vi "Position First Tab Button.vi"(7 "TabCtl Refnum":refnum<vi>, 8 "error in (no error)":errorcluster, 11 "Button Ref":refnum<vi>) -> (0 "error out":errorcluster)   [LabVIEW 2014]
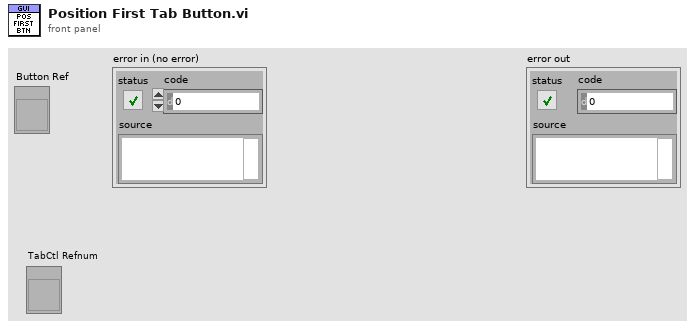
[diagram p1: front panel]
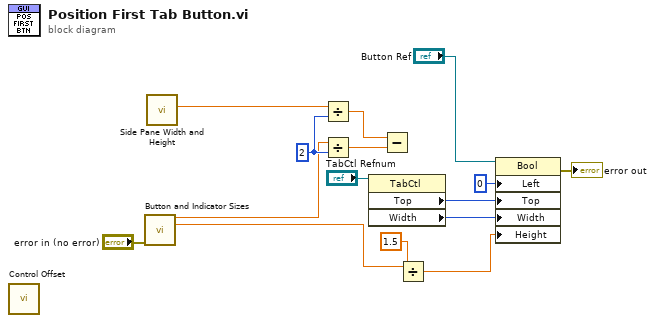
[diagram p0: block diagram]
diagram:
  w6 = u32 2 ("y")
  n1 = call "Control Offset.vi"() -> ()  [unwired: 11 in, 1 out]
  n2 = call "Button and Indicator Sizes.vi"("error in (no error)"="error in (no error)") -> ("Button Width"=w3:dbl, "Button Height"=w12:dbl)  [unwired: 10 in, 3 out]
  n3 = call "Side Pane Width and Height.vi"() -> ("Width"=w4:dbl)  [unwired: 9 in, 2 out]
  n4 = Divide(x=w4, y=w6) -> (x/y=w7:dbl)
  n5 = Divide(x=w3, y=w6) -> (x/y=w5:dbl)
  n6 = property class="TabCtl"(reference="TabCtl Refnum") -> ("Top"=w8:i32, "Width"=w2:u32)  [unwired: 1 in, 2 out]
  n7 = Subtract(x=w7, y=w5) -> ()  [unwired: 1 out]
  n8 = Divide(x=w12, y=1.5) -> (x/y=w10:dbl)
  n9 = property class="Bool"(reference="Button Ref", "Left"=0 ("Position:Left"), "Top"=w8, "Width"=w2, "Height"=w10) -> (error out=→"error out":errorcluster)  [unwired: 1 in, 1 out]
